vi "SetInitTime.vi"() -> ()   [LabVIEW 2019]
panel:
  out "seconds since 1Jan1904":timestamp
  in  "Ring":u16(ring) items=["Init", "Read"]
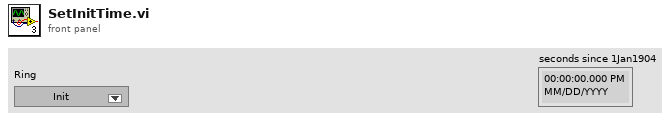
[diagram p1: front panel]
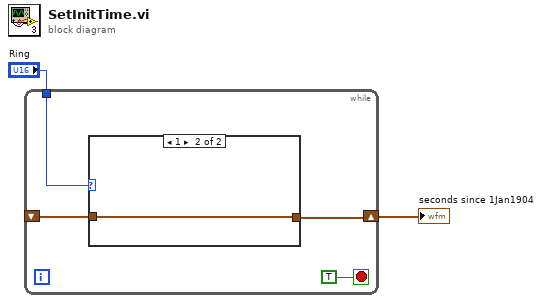
[diagram p0: block diagram]
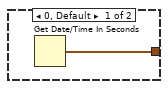
[diagram p2: hidden frame]
diagram:
  n1 = while {
    tunnel: "Ring" -> [w5]
    shift-right: [w4] -> w1
    shift-left: _ -> [w3]
    stop <- TRUE stop-if-true
    n2 = case shown="1" w5 {
      tunnel: [w7 w8] -> w4
      tunnel: w3 -> [_ w8]
      frame 0, Default {
        n3 = Get Date/Time In Seconds() -> (seconds since 1Jan1904=w7:timestamp)
      }
      frame 1 {
      }
    }
  }
  "seconds since 1Jan1904" <- w1
